vi "Abort Generation.vi"(8 "error in (no error)":errorcluster, 11 "CS++Fgen in":refnum<class "CS++Fgen.lvclass">) -> (0 "error out":errorcluster, 3 "CS++Fgen out":refnum<class "CS++Fgen.lvclass">)   [LabVIEW 2013, in "CS++Fgen.lvlib" / "CS++Fgen.lvclass"]
doc: "This VI aborts a previously initiated signal generation. If the function generator is in the Output Generation State, this VI moves the function generator to the Configuration State. If the function generator is already in the Configuration State, the VI does nothing.\n\nYou can configure the output of the function generator regardless of whether the function generator is in the Configuration State or the Generation State. This means that you are not required to call the IviFgen Abort Generation VI prior to configuring the output of the function generator. \n\nMany function generators constantly generate an output signal, and do not require you to abort signal generation prior to configuring the instrument. If a function generator's output cannot be aborted (i.e., the function generator cannot stop generating a signal) this function does nothing.\n\nYou are not required to call the IviFgen Initiate Generation and IviFgen Abort Generation VIs. Whether you choose to call these VIs in an application program has no impact on interchangeability. You can choose to use these VIs if you want to optimize your application for instruments that exhibit increased performance when output configuration is performed while the instrument is not generating a signal.\n\nNotes:\n\n(1) This VI does not normally check the instrument status. Typically, you call this VI only in a sequence of calls to other low-level driver VIs. The sequence performs one operation. You use the low-level VIs to optimize one or more aspects of interaction with the instrument. If you want to check the instrument status, call the IviFgen Error-Query VI at the conclusion of the sequence."
uses:
  CS++Fgen.lvclass
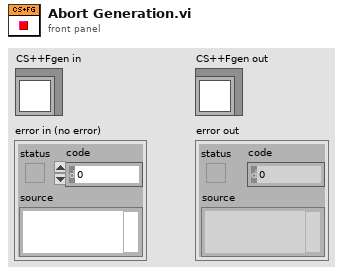
[diagram p1: front panel]
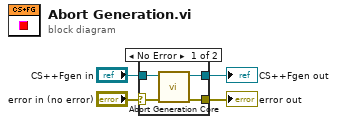
[diagram p0: block diagram]
diagram:
  n1 = case shown="No Error" "error in (no error)" {
    selector: "error in (no error)" -> [w6 w10]
    tunnel: [w5 w10] -> w3
    tunnel: [w7 w9] -> w1
    tunnel: "CS++Fgen in" -> [w8 w9]
    frame No Error {
      n2 = call-dynamic "Abort Generation Core.vi"("error in (no error)"=w6, "CS++Fgen in"=w8) -> ("error out"=w5:errorcluster, "CS++Fgen out"=w7:refnum<class "CS++Fgen.lvclass">)  [unwired: 8 in]
    }
    frame Error {
    }
  }
  "error out" <- w3
  "CS++Fgen out" <- w1
